vi "Pneumatic_Command_Get_Tele.vi"(11 "RT FIFO":u64) -> (2 "Status":T2, 3 "Cluster Out":T1)   [LabVIEW 2015]
uses:
  <userlib>/836-Library/Pneumatics/Support_Code/Pneumatics_Notifier.ctl
  <userlib>/836-Library/Pneumatics/Support_Code/Pneumatics_Command.ctl
  <userlib>/836-Library/Pneumatics/Support_Code/Pneumatics_Status.ctl
panel:
  in  "Cluster":T1
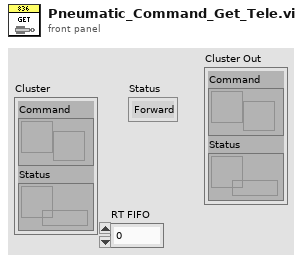
[diagram p1: front panel]
types:
  T1 = typedef "Pneumatics_Notifier.ctl" = cluster{"Command":refnum<notifier>, "Status":refnum<queue>}
  T2 = typedef "Pneumatics_Status.ctl" = enum16{"Forward", "Reverse", "Moving"}
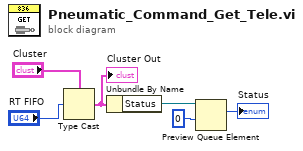
[diagram p0: block diagram]
diagram:
  n1 = Type Cast(type="Cluster", x="RT FIFO") -> (*(type *) &x=w1:T1)
  "Cluster Out" <- w1
  n2 = Unbundle By Name(w1) -> ("Status"=w6:refnum<queue>)
  n3 = Preview Queue Element(queue=w6, timeout in ms (-1)=0) -> (element=→"Status":T2)  [unwired: 1 in, 3 out]
